vi "Measuring R with Agilent 34401A.vi"() -> ()   [LabVIEW 2018]
uses:
  <instrlib>/Agilent 34401/Public/Data/Read (Single Point).vi
  <instrlib>/Agilent 34401/Agilent 34401.lvlib
panel:
  in  "Function (0: DC Voltage)":u16(ring)=2 items=["DC Voltage", "AC Voltage", "2 - Wire Resistance", "4 - Wire Resistance", "DC Current", "AC Current", "Frequency", "Period", "Continuity", "Diode Checking", "VDC:VDC Ratio", "Temperature", "Capacitance"]
  in  "stop":bool
  out "Measurement":dbl format="%_6p"
  in  "VISA resource name":refnum<visa-resource-name>
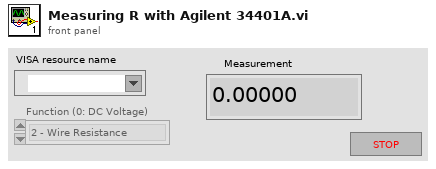
[diagram p1: front panel]
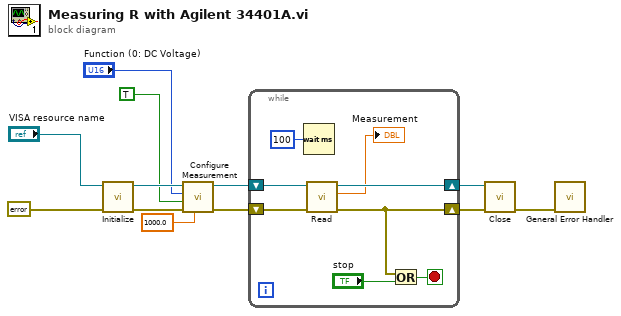
[diagram p0: block diagram]
diagram:
  n1 = call <instrlib>:"Initialize.vi"("error in (no error)"=errorcluster {"status"=FALSE, "code"=0, "source"=""}, "VISA resource name"="VISA resource name") -> ("error out"=w10:errorcluster, "VISA resource name out"=w9:refnum<visa-resource-name>)  [unwired: 8 in]
  n2 = call <instrlib>:"Configure Measurement.vi"("Manual Range (1.00)"=1000.0, "error in (no error)"=w10, "Enable Auto Range (T: Enable)"=TRUE, "Function (0: DC Voltage)"="Function (0: DC Voltage)", "VISA resource name"=w9) -> ("error out"=w2:errorcluster, "VISA resource name out"=w1:refnum<visa-resource-name>)  [unwired: 5 in]
  n3 = while {
    shift-right: [w13] -> w6
    shift-left: w2 -> [w20]
    shift-right: [w18] -> w7
    shift-left: w1 -> [w19]
    stop <- w14 stop-if-true
    n4 = Wait (ms)(milliseconds to wait=u32 100) -> ()  [unwired: 1 out]
    n5 = call-poly <instrlib>:"Read.vi"("error in (no error)"=w20, "VISA resource name"=w19) -> ("error out"=w13:errorcluster, "Measurement"=→"Measurement":dbl, "VISA resource name out"=w18:refnum<visa-resource-name>)  [unwired: 7 in]
    n6 = Or(x=w13, y="stop") -> (x .or. y?=w14:bool)
  }
  n7 = call <instrlib>:"Close.vi"("error in (no error)"=w6, "VISA resource name"=w7) -> ("error out"=w3:errorcluster)  [unwired: 9 in]
  n8 = call <vilib>:"General Error Handler.vi"("error in (no error)"=w3) -> ()  [unwired: 10 in, 5 out]
